vi "Indicator_Color.vi"(11 "Color Selector":T2) -> (3 "Text Colors":T1)   [LabVIEW 2019, in "Base Software.lvlib" / "Main.lvlib" / "Base Software.lvclass"]
uses:
  Project/Base Software.lvclass
  Custom Controls/Color_Items.ctl
  <vilib>/Utility/miscctls.llb/LVTextColorsTypeDef.ctl
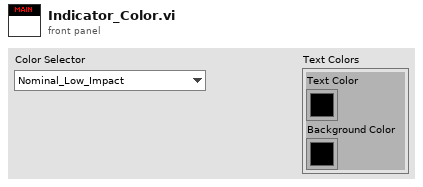
[diagram p1: front panel]
types:
  T1 = typedef "LVTextColorsTypeDef.ctl" = cluster{"Text Color":u32, "Background Color":u32}
  T2 = typedef "Base Software.lvlib/Main.lvlib/Base Software.lvclass/Color_Items.ctl" = enum16{"Nominal_Low_Impact", "Nominal", "User_Interaction", "Warning", "Error"}
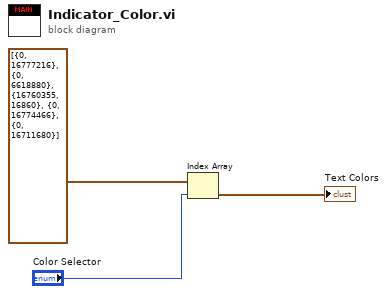
[diagram p0: block diagram]
diagram:
  n1 = Index Array(array=cluster{"Color Box":u32, "Color Box 2":u32}[] [{"Color Box"=0, "Color Box 2"=16777216}, {"Color Box"=0, "Color Box 2"=6618880}, {"Color Box"=16760355, "Color Box 2"=16860}, {"Color Box"=0, "Color Box 2"=16774466}, {"Color Box"=0, "Color Box 2"=16711680}] ("Array"), index="Color Selector") -> (element=→"Text Colors":cluster{"Color Box":u32, "Color Box 2":u32})
